vi "Get Message Type.vi"(8 "error in":errorcluster, 11 "message or subaddress":T2 format="%.0x") -> (0 "error out":errorcluster, 2 "message type":T1, 3 "message or subaddress out":T2 format="%.0x", 4 "found?":bool)   [LabVIEW 2020, in "AIM MIL-STD-1553 Scripting.lvlib"]
doc: "Returns the <b>message type</b> of the input <b>message or subaddress</b>."
uses:
  AIM MIL-STD-1553 Scripting.lvlib
  <vilib>/NI VeriStand/Custom Device API/Custom Device Item Ref.ctl
  Shared/Message Type.ctl
  Constants.vi
  <vilib>/NI VeriStand/Custom Device API/Get Item Property (String).vi
  <vilib>/NI VeriStand/Custom Device API/Custom Device API.lvlib
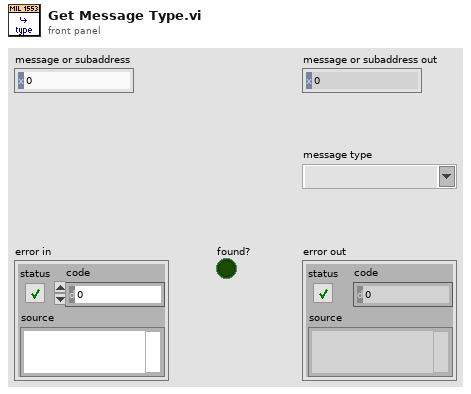
[diagram p1: front panel]
types:
  T1 = typedef "Message Type.ctl" = string
  T2 = typedef "Custom Device API.lvlib/Custom Device Item Ref.ctl" = u64
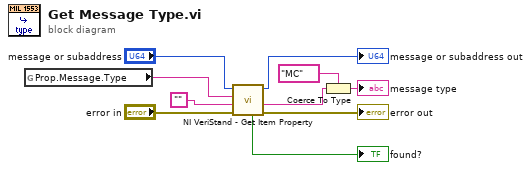
[diagram p0: block diagram]
diagram:
  n1 = global read "Constants.vi" "Prop.Message.Type"() -> (w5:string)
  n2 = call-poly <vilib>:"NI VeriStand - Get Item Property.vi"("error in (no error)"="error in", "Default Value"="", "Property Name"=w5, "Item Ref in"="message or subaddress") -> ("error out"=→"error out":errorcluster, "Value"=w2:string, "Item Ref out"=→"message or subaddress out":T2, "Found?"=→"found?":bool)  [unwired: 4 in]
  n3 = Coerce To Type(0:w2, 1:T1 "MC" ("message type")) -> (2:→"message type":T1)
